vi "carga_dc_load_capacidade.vi"() -> ()   [LabVIEW 2016]
panel:
  in  "Capacidade":dbl
  out "DC Voltage":dbl caption="measured value" format="%#.4f"
  out "DC Current":dbl caption="measured value" format="%#.4f"
  in  "stop":bool
  out "CC Active":bool
  in  "Current Enabled":bool caption="Set Current"
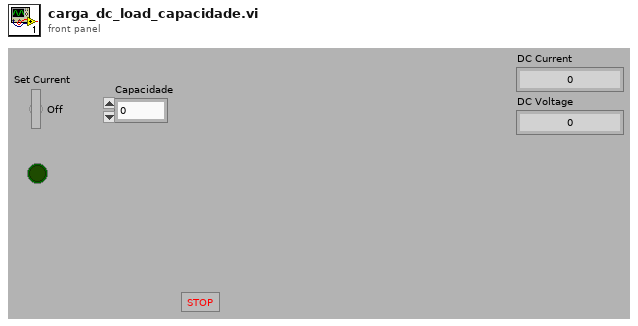
[diagram p1: front panel]
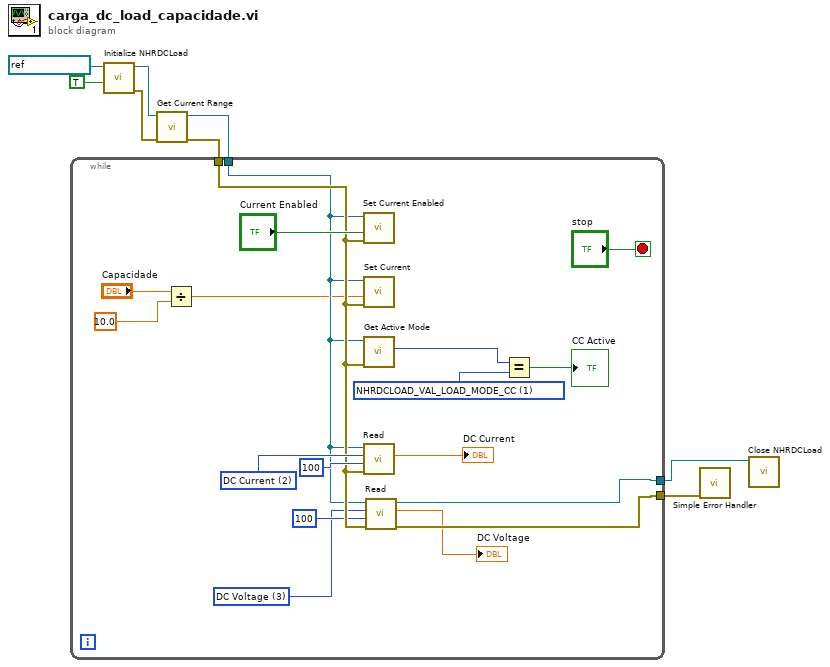
[diagram p0: block diagram]
diagram:
  n1 = call <instrlib>:"Initialize NHRDCLoad.vi"("reset device (Off)"=TRUE, "resource name"=refnum<visa-resource-name> "DC Load 1") -> ("error out"=w4:errorcluster, "instrument handle out"=w6:refnum<visa-resource-name>)  [unwired: 8 in]
  n2 = call <instrlib>:"Get Current Range.vi"("error in (no error)"=w4, "instrument handle"=w6) -> ("error out"=w3:errorcluster, "instrument handle out"=w5:refnum<visa-resource-name>)  [unwired: 7 in, 1 out]
  n3 = while {
    tunnel: w5 -> [w18]
    tunnel: w3 -> [w19]
    tunnel: [w16] -> w2
    tunnel: [w17] -> w1
    stop <- "stop" stop-if-true
    w14 = u16 3 items=["AC + DC Current", "AC + DC Voltage", "DC Current", "DC Voltage", "First 10% Current", "First 10% Voltage", "Last 10% Current", "Last 10% Voltage", "Negative Peak Current", "Negative Peak Voltage", "Positive Peak Current", "Positive Peak Voltage", "Average Power", "Resistance", "RMS Current", "RMS Voltage"] ("Measurement")
    w21 = u16 2 items=["AC + DC Current", "AC + DC Voltage", "DC Current", "DC Voltage", "First 10% Current", "First 10% Voltage", "Last 10% Current", "Last 10% Voltage", "Negative Peak Current", "Negative Peak Voltage", "Positive Peak Current", "Positive Peak Voltage", "Average Power", "Resistance", "RMS Current", "RMS Voltage"] ("Measurement")
    w20 = 1 items=["NHRDCLOAD_VAL_LOAD_MODE_OFF"=0, "NHRDCLOAD_VAL_LOAD_MODE_CC"=1, "NHRDCLOAD_VAL_LOAD_MODE_CR"=2, "NHRDCLOAD_VAL_LOAD_MODE_CV"=4, "NHRDCLOAD_VAL_LOAD_MODE_CP"=8, "NHRDCLOAD_VAL_LOAD_MODE_XCC"=16, "NHRDCLOAD_VAL_LOAD_MODE_LED"=32, "NHRDCLOAD_VAL_LOAD_MODE_MPPT"=64, "NHRDCLOAD_VAL_LOAD_MODE_XY"=128, "NHRDCLOAD_VAL_LOAD_MODE_SC"=32768] ("active mode")
    n4 = Divide(x="Capacidade", y=10.0) -> (x/y=w9:dbl)
    n5 = call <instrlib>:"Set Current Enabled.vi"("error in (no error)"=w19, "current enabled (false)"="Current Enabled", "instrument handle"=w18) -> ()  [unwired: 7 in, 2 out]
    n6 = call <instrlib>:"Set Current.vi"("error in (no error)"=w19, "current (0.0)"=w9, "instrument handle"=w18) -> ()  [unwired: 7 in, 2 out]
    n7 = call <instrlib>:"Get Active Mode.vi"("error in (no error)"=w19, "instrument handle"=w18) -> ("active mode"=w25:i32)  [unwired: 7 in, 2 out]
    n8 = call <instrlib>:"Read.vi"("error in (no error)"=w19, "max time milliseconds (infinite)"=100, "measurement (NHRDCLOAD_VAL_MEASURE_AC_PLUS_DC_CURRENT)"=w21, "instrument handle"=w18) -> ("measured value"=→"DC Current":dbl)  [unwired: 5 in, 2 out]
    n9 = call <instrlib>:"Read.vi"("error in (no error)"=w19, "max time milliseconds (infinite)"=100, "measurement (NHRDCLOAD_VAL_MEASURE_AC_PLUS_DC_CURRENT)"=w14, "instrument handle"=w18) -> ("error out"=w16:errorcluster, "measured value"=→"DC Voltage":dbl, "instrument handle out"=w17:refnum<visa-resource-name>)  [unwired: 5 in]
    n10 = Equal?(x=w25, y=w20) -> (x = y?=→"CC Active":bool)
  }
  n11 = call <vilib>:"Simple Error Handler.vi"("error in (no error)"=w2) -> ()  [unwired: 4 in, 5 out]
  n12 = call <instrlib>:"Close NHRDCLoad.vi"("instrument handle"=w1) -> ()  [unwired: 10 in, 1 out]
